vi "MagX Get Status.vi"(6 "Update experiment info file":bool, 7 "url":string, 8 "error in":errorcluster, 11 "Experiment ID":string="Cell_3") -> (0 "error out":errorcluster, 3 "Data out":cluster{"user":string, "expid":string})   [LabVIEW 2021]
uses:
  7bf855a0-2889-4335-a077-b20b33b30227.vi
  <vilib>/JDP Science/JSONtext/JSON text to Variant.vi
  <vilib>/JDP Science/JSONtext/LVClass Serializer/JSONtext LVClass Serializer.lvclass
  <vilib>/httpClient/LabVIEWHTTPClient.lvlib
panel:
  in  "Experiment info file":path=path "C:/Data/experiment_info.txt"
  out "body":string
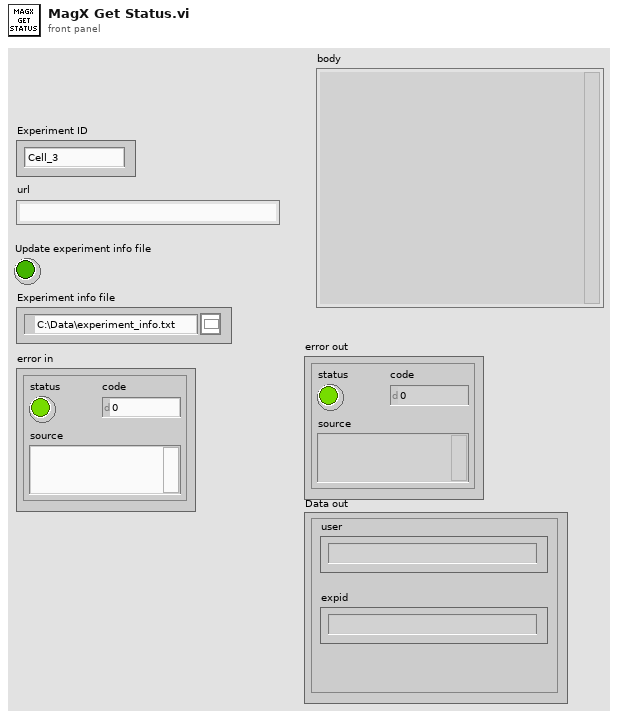
[diagram p1: front panel]
types:
  T1 = typedef "LabVIEWHTTPClient.lvlib/ClientHandle.ctl" = refnum<k1>
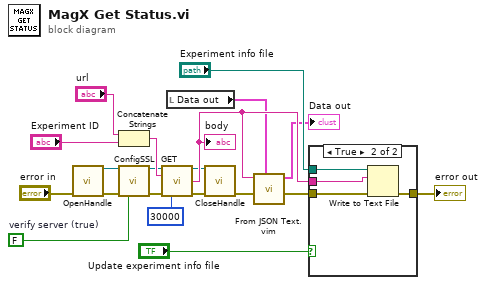
[diagram p0: block diagram]
diagram:
  w8 = FALSE  # verify server (true)
  n1 = call <vilib>:"OpenHandle.vi"("error in (no error)"="error in") -> ("client handle out"=w12:T1, "error out"=w11:errorcluster)  [unwired: 13 in]
  n2 = Concatenate Strings("url", "Experiment ID") -> (w19:string)
  n3 = call <vilib>:"ConfigSSL.vi"("client handle"=w12, "error in (no error)"=w11, "verify server (true)"=w8) -> ("client handle out"=w9:T1, "error out"=w10:errorcluster)  [unwired: 11 in]
  n4 = call <vilib>:"GET.vi"("client handle"=w9, "url"=w19, "error in (no error)"=w10, "timeout (10000)"=30000) -> ("client handle out"=w2:T1, "body"=w13:string, "error out"=w3:errorcluster)  [unwired: 8 in, 1 out]
  "body" <- w13
  n5 = local read "Data out"() -> (w6:cluster{"user":string, "expid":string})
  n6 = call <vilib>:"CloseHandle.vi"("client handle"=w2, "error in (no error)"=w3) -> ("error out"=w4:errorcluster)  [unwired: 13 in]
  n7 = call "From JSON Text.vim"("Data Type and Default Value"=w6, "error in (no error)"=w4, "JSON"=w13) -> ("error out"=w15:errorcluster, "Data out"=→"Data out":cluster{"user":string, "expid":string})  [unwired: 7 in]
  n8 = case shown="True" "Update experiment info file" {
    tunnel: w15 -> [w21 w25]
    tunnel: "Experiment info file" -> [_ w24]
    tunnel: [w21 w23] -> w5
    tunnel: w13 -> [_ w22]
    frame False {
    }
    frame True {
      n9 = Write to Text File(file (use dialog)=w24, text=w22, error in=w25) -> (error out=w23:errorcluster)  [unwired: 1 in, 2 out]
    }
  }
  "error out" <- w5
